vi "getROI.vi"(11 "CamSettings":T1) -> (3 "ROI":i32[][](array[numeric]))   [LabVIEW 2020]
uses:
  CamSettings_Typdef.ctl
  CamSettingSUB_TypDEf.ctl
  MagAnalysis_Online_Bella/SubVis/CamAndObj_TypDEf.ctl
  shared/OnOffTypeDef.ctl
  userROI.ctl
  shared/numericVariable_TypeDef.ctl
  CamRoiTypDef.ctl
  BaseDriver/BaseDriver.lvclass
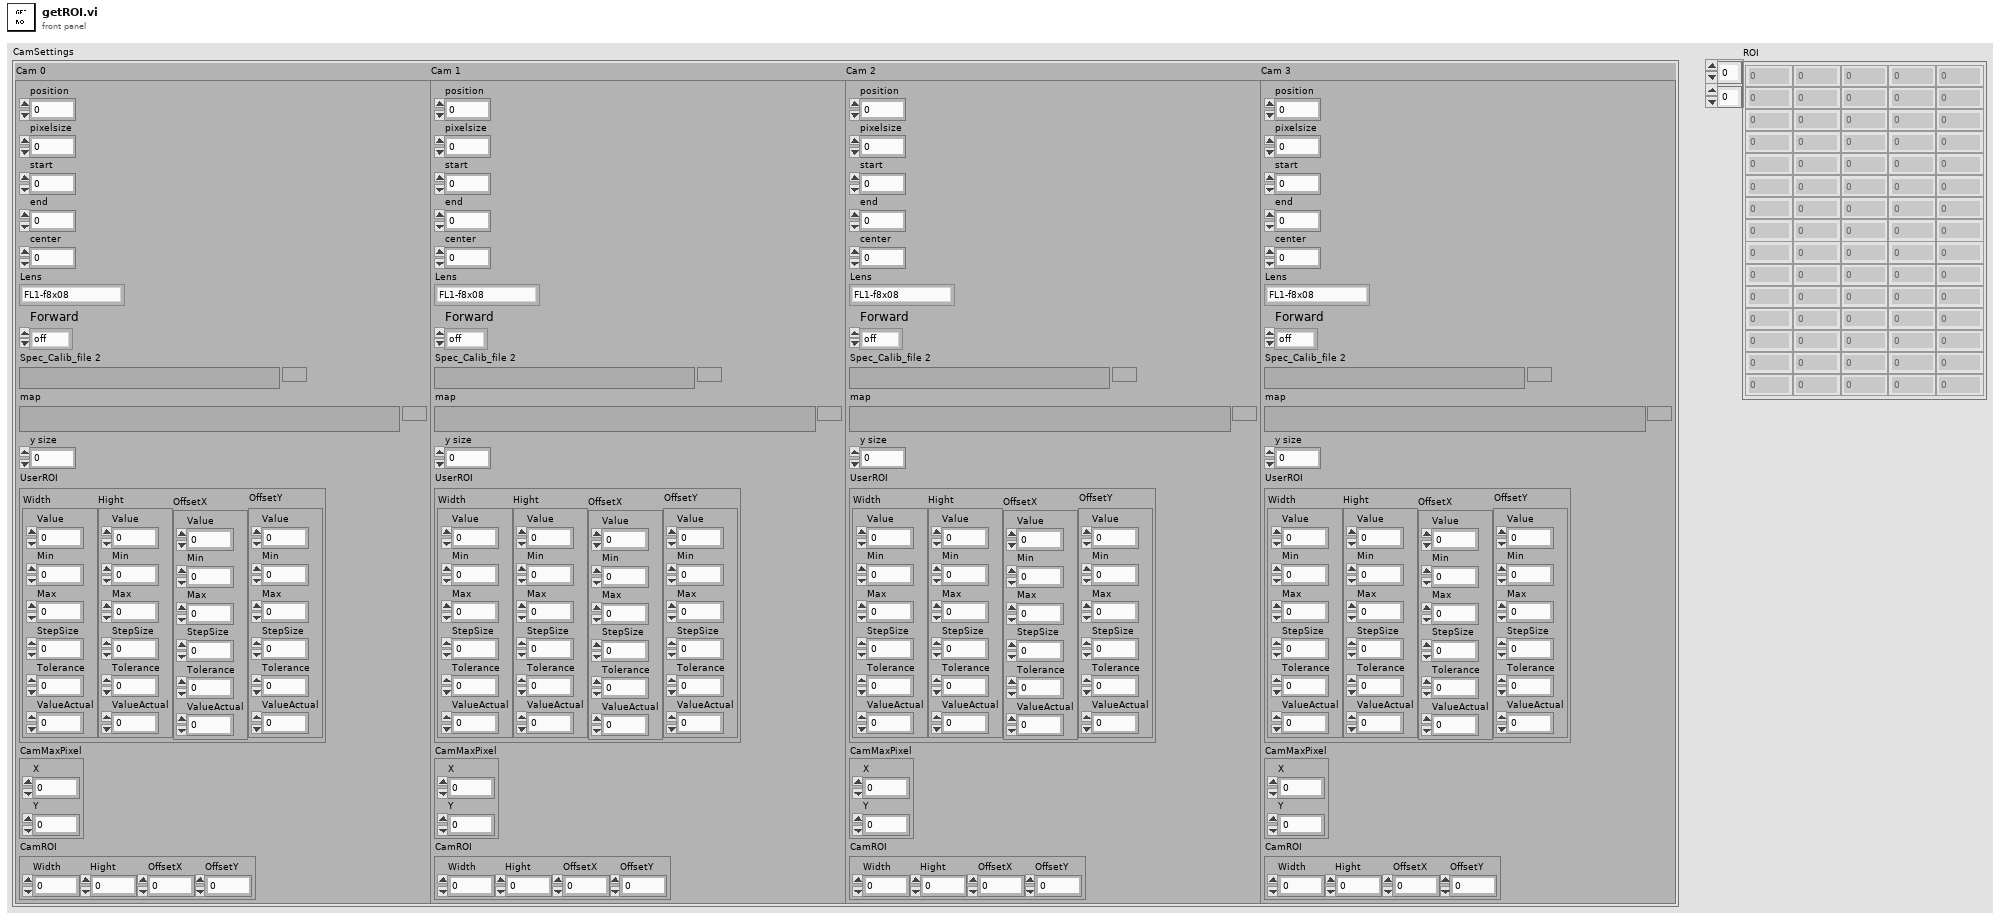
[diagram p1: front panel]
types:
  T1 = typedef "CamSettings_Typdef.ctl" = cluster{"Cam 0":T2, "Cam 1":T2, "Cam 2":T2, "Cam 3":T2}
  T2 = typedef "CamSettingSUB_TypDEf.ctl" = cluster{"position":dbl, "pixelsize":dbl, "start":dbl, "end":dbl, "center":dbl, "Lens":T3, "Forward":T4, "Spec_Calib_file 2":path, "map":path, "y size":i32, "UserROI":T5, "CamMaxPixel":cluster{"X":i32, "Y":i32}, "CamROI":T7}
  T3 = typedef "CamAndObj_TypDEf.ctl" = enum16{"FL1-f8x08", "FL1-f8x06", "FL1-f8", "ch300-f50", "FL2G-f8", "FL3M14-f8", "FL3M14-f8x08", "FL3M14-f8x08(2x2)"}
  T4 = typedef "OnOffTypeDef.ctl" = enum16{"off", "on"}
  T5 = typedef "userROI.ctl" = cluster{"Width":T6, "Hight":T6, "OffsetX":T6, "OffsetY":T6}
  T6 = typedef "BaseDriver.lvclass/numericVariable_TypeDef.ctl" = cluster{"Value":dbl, "Min":dbl, "Max":dbl, "StepSize":dbl, "Tolerance":dbl, "ValueActual":dbl}
  T7 = typedef "CamRoiTypDef.ctl" = cluster{"Width":dbl, "Hight":dbl, "OffsetX":dbl, "OffsetY":dbl}
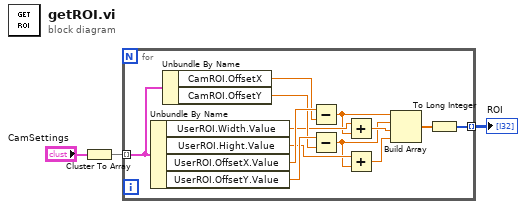
[diagram p0: block diagram]
diagram:
  n1 = Cluster To Array(cluster="CamSettings") -> (array=w2:T2[])
  n2 = for {
    tunnel: w2 -> [w15] mode=indexing
    tunnel: [w16] -> w1 mode=indexing
    n3 = Unbundle By Name(w15) -> ("UserROI.Width.Value"=w10:dbl, "UserROI.Hight.Value"=w7:dbl, "UserROI.OffsetX.Value"=w14:dbl, "UserROI.OffsetY.Value"=w12:dbl)
    n4 = Unbundle By Name(w15) -> ("CamROI.OffsetX"=w13:dbl, "CamROI.OffsetY"=w11:dbl)
    n5 = Subtract(x=w14, y=w13) -> (x-y=w9:dbl)
    n6 = Subtract(x=w12, y=w11) -> (x-y=w6:dbl)
    n7 = Add(x=w10, y=w9) -> (x+y=w8:dbl)
    n8 = Add(x=w7, y=w6) -> (x+y=w5:dbl)
    n9 = Build Array(w9, w6, w8, w5) -> (w4:dbl[])
    n10 = To Long Integer(number=w4) -> (32bit integer=w16:i32[])
  }
  "ROI" <- w1
